vi "random insert.vi"(6 "empty rounds":u32, 7 "live rounds":u32) -> (1 "chamber":i32[](array[numeric]))   [LabVIEW 2025]
uses:
  4801f10c-0daa-45ec-b7f4-2c5e7cf59321.vi
  636b7669-5195-4fe2-9d9a-1106ac0c26aa.vi
  b591cb89-e3bc-4ada-b7d8-20f44477c02e.vi
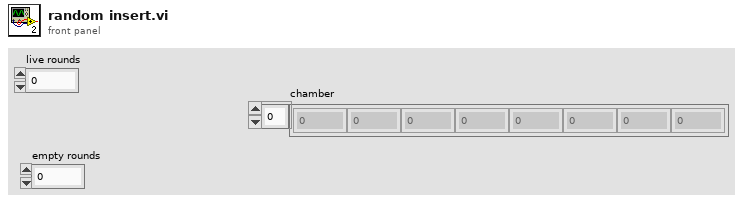
[diagram p1: front panel]
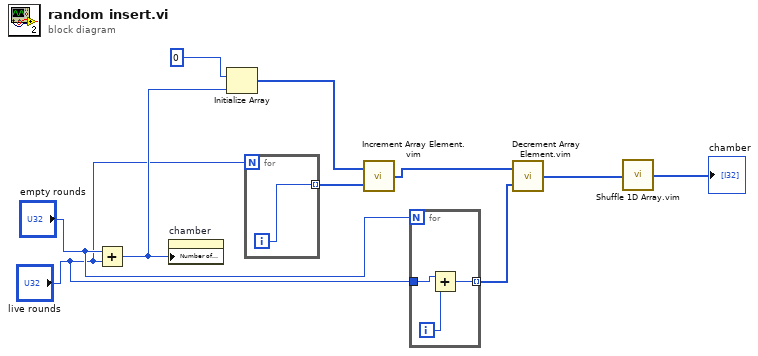
[diagram p0: block diagram]
diagram:
  n1 = Add(x="empty rounds", y="live rounds") -> (x+y=w9:u32)
  n2 = property on="chamber" class="Arr (strict)"("Number of Columns"=w9) -> ()  [unwired: 2 in, 2 out]
  n3 = Initialize Array(0, w9) -> (w8:i32[])
  n4 = for {
    N: "live rounds" -> [_]
    tunnel: [w11] -> w7 mode=indexing
    i -> [w11]
  }
  n5 = call "Increment Array Element.vim"("index"=w7, "array in"=w8) -> ("array out"=w5:i32[])
  n6 = for {
    N: "empty rounds" -> [_]
    tunnel: "live rounds" -> [w13]
    tunnel: [w12] -> w3 mode=indexing
    i -> [w14]
    n7 = Add(x=w13, y=w14) -> (x+y=w12:u32)
  }
  n8 = call "Decrement Array Element.vim"("index"=w3, "array in"=w5) -> ("array out"=w2:i32[])
  n9 = call "Shuffle 1D Array.vim"("array"=w2) -> ("shuffled array"=→"chamber":i32[])  [unwired: 4 in]
